vi "Read UI Refnum.vi"(8 "error in (no error)":errorcluster, 11 "ConfigureableObject in":refnum<class "CallEXEStep.lvclass">) -> (0 "error out":errorcluster, 2 "VI Refnum":refnum<vi>, 3 "ConfigureableObject out":refnum<class "CallEXEStep.lvclass">)   [LabVIEW 2015, in "CallEXEStep.lvclass"]
uses:
  CallEXEStep.lvclass
  EXEStep Configure UI.vi
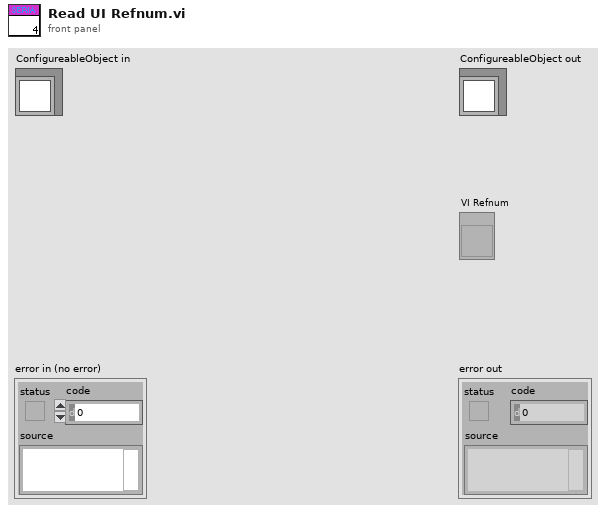
[diagram p1: front panel]
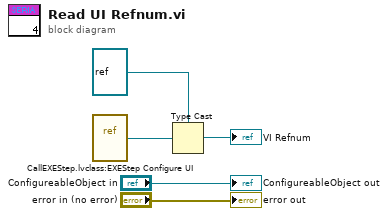
[diagram p0: block diagram]
diagram:
  n1 = vi-ref "CallEXEStep.lvclass:EXEStep Configure UI.vi"() -> (w5:refnum<vi>)
  n2 = Type Cast(type=refnum<vi> refnum ("vi reference"), x=w5) -> (*(type *) &x=→"VI Refnum":refnum<vi>)
  "error out" <- "error in (no error)"
  "ConfigureableObject out" <- "ConfigureableObject in"
